vi "Multiple Notifiers.vi"(6 "Method":T2(ring), 8 "error in (no error)":errorcluster, 9 "Functions":enum16{"Raw data", "Other data"}(ring)) -> (0 "error out":errorcluster, 2 "element":refnum<notifier>)   [LabVIEW 2020]
uses:
  Def/Notifier_Def.ctl
panel:
  in  "Notifier_Data":T1
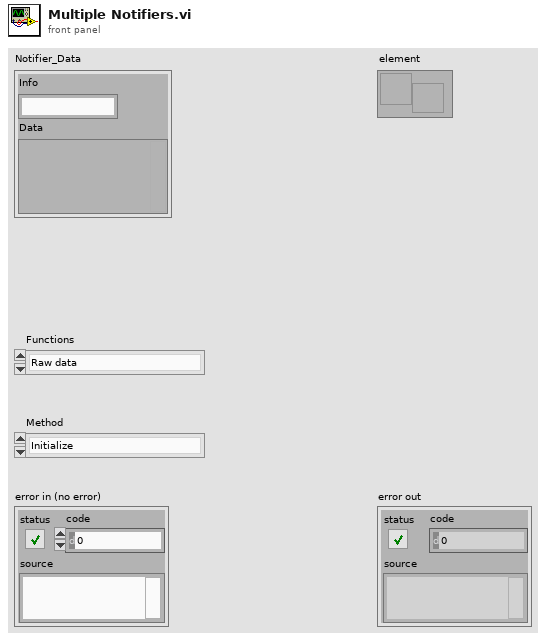
[diagram p1: front panel]
types:
  T1 = typedef "Notifier_Def.ctl" = cluster{"Info":string, "Data":variant}
  T2 = enum16{"Initialize", "Write", "Read", "Release All Notifiers"}
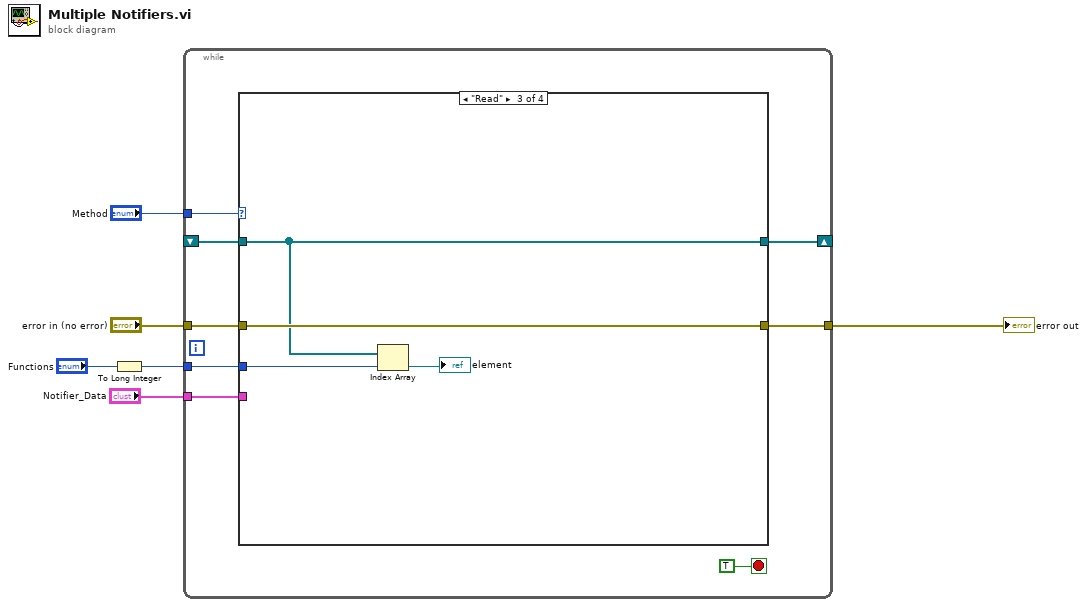
[diagram p0: block diagram]
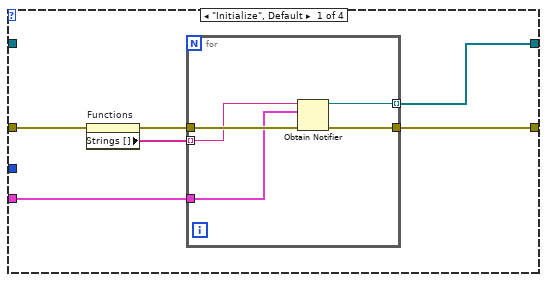
[diagram p2: hidden frame]
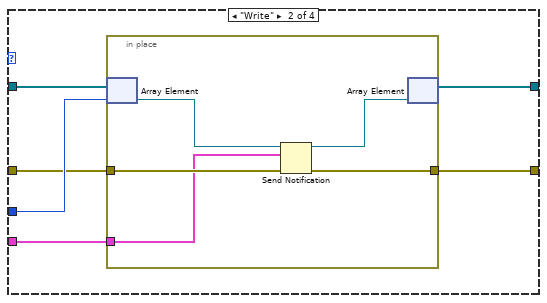
[diagram p3: hidden frame]
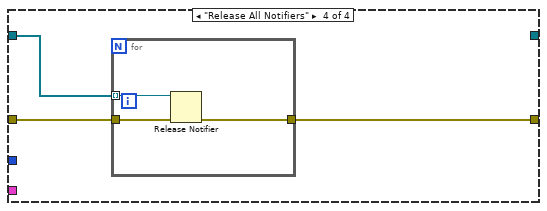
[diagram p4: hidden frame]
diagram:
  n1 = To Long Integer(number="Functions") -> (32bit integer=w1:i32)
  n2 = while {
    tunnel: "error in (no error)" -> [w13]
    tunnel: "Notifier_Data" -> [w12]
    tunnel: [w11] -> w4
    tunnel: "Method" -> [w10]
    shift-right: [w9] -> _
    shift-left: _ -> [w8]
    tunnel: w1 -> [w7]
    stop <- TRUE stop-if-true
    n3 = case shown="\"Read\"" w10 {
      tunnel: w13 -> [w18 w29 w39 w42]
      tunnel: w12 -> [w20 w27 _ _]
      tunnel: [w19 w28 w39 w41] -> w11
      tunnel: [w15 w26 w38 _] -> w9
      tunnel: w8 -> [_ w31 w38 w43]
      tunnel: w7 -> [_ w30 w40 _]
      frame "Initialize", Default {
        n4 = property on="Functions" class="Enum (strict)"(error in=w18) -> (error out=w17:errorcluster, "Strings []"=w16:string[])  [unwired: 1 in, 1 out]
        n5 = for {
          tunnel: w17 -> [w25]
          tunnel: w20 -> [w24]
          tunnel: [w23] -> w19
          tunnel: w16 -> [w22] mode=indexing
          tunnel: [w21] -> w15 mode=indexing
          n6 = Obtain Notifier(name (unnamed)=w22, notification data type=w24, error in (no error)=w25) -> (notifier out=w21:refnum<notifier>, error out=w23:errorcluster)  [unwired: 1 in, 1 out]
        }
      }
      frame "Write" {
        n7 = in-place {
          in-place-border: w29 -> [w35]
          in-place-border: [w34] -> w28
          in-place-border: w27 -> [w32]
          n8 = in-place-array #1(w31, w30) -> (w36:refnum<notifier>)
          n9 = Send Notification(notification=w32, notifier=w36, error in (no error)=w35) -> (notifier out=w33:refnum<notifier>, error out=w34:errorcluster)
          n10 = in-place-array #1(w33) -> (w26:refnum<notifier>[])  [unwired: 1 out]
        }
      }
      frame "Read" {
        n11 = Index Array(array=w38, index=w40) -> (element=→"element":refnum<notifier>)
      }
      frame "Release All Notifiers" {
        n12 = for {
          tunnel: w43 -> [w46] mode=indexing
          tunnel: w42 -> [w45]
          tunnel: [w44] -> w41
          n13 = Release Notifier(notifier=w46, error in (no error)=w45) -> (error out=w44:errorcluster)  [unwired: 1 in, 2 out]
        }
      }
    }
  }
  "error out" <- w4
